vi "Power up time PWM rw.vi"(5 "INDEX":enum16{"Read", "Write"}(ring), 7 "IP":string="192.168.23.100", 8 "error in (no error)":errorcluster, 9 "PWR UP TIME(ms)":u16(knob)=5 min=5 max=2000 step=1 scale=5.0..2000.0, 10 "PORT":dbl=1.0 min=1.0 max=4.0 step=1.0, 11 "MASTER":dbl=1.0 min=1.0 max=10.0 step=1.0) -> (0 "error out":errorcluster, 2 "Startup time":u32 format="%^#.10g ms")   [LabVIEW 2022 SP3]
uses:
  <vilib>/NI/Advanced HTTP Client/POST (Buffer).vi
  <vilib>/NI/Advanced HTTP Client/Session.lvclass
panel:
  out "JSON STRING PAYLOAD":string
  # "SMART conn PWM start Read /Write"
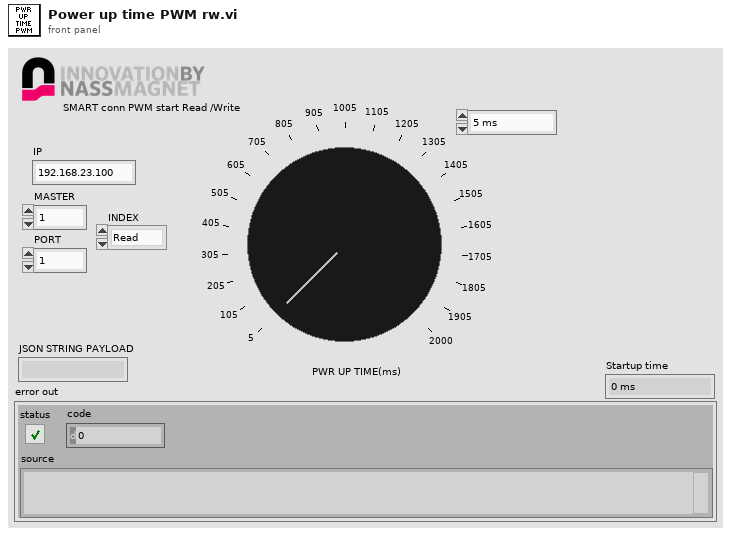
[diagram p1: front panel]
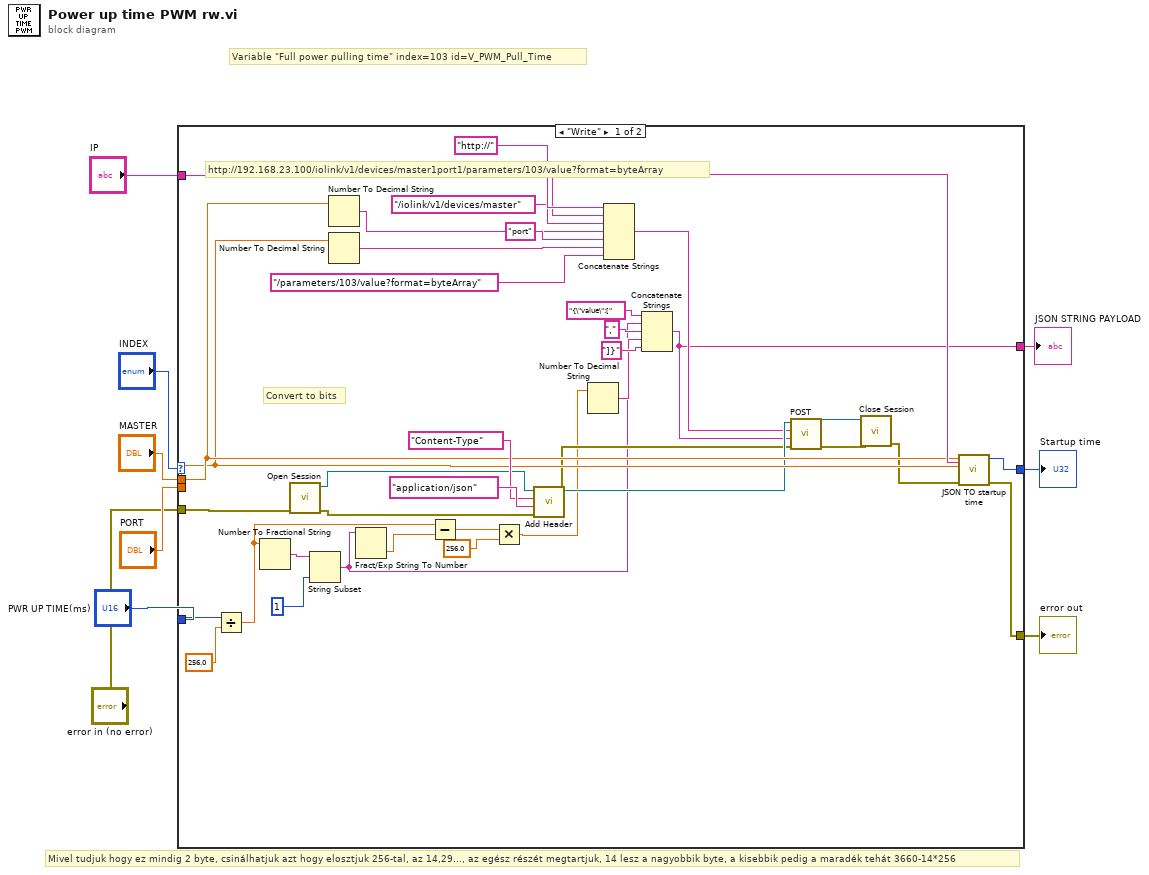
[diagram p0: block diagram]
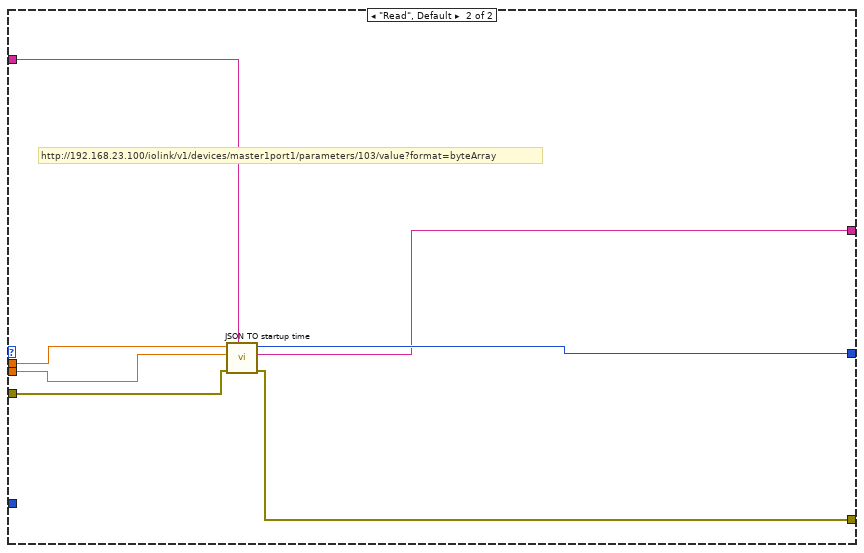
[diagram p2: hidden frame]
diagram:
  # "Variable \"Full power pulling time\" index=103 id=V_PWM_Pull_Time"
  # "Mivel tudjuk hogy ez mindig 2 byte, csinálhatjuk azt hogy elosztjuk 256-tal, az 14,29..., az egész részét megtartjuk, 14 lesz a nagyobbik byte, a kisebbik pedig a maradék tehát 3660-14*256"
  n1 = case shown="\"Write\"" "INDEX" {
    tunnel: "MASTER" -> [w33 w49]
    tunnel: "PORT" -> [w32 w53]
    tunnel: "IP" -> [w36 w52]
    tunnel: [w46 w51] -> w6
    tunnel: [w45 w50] -> w5
    tunnel: "error in (no error)" -> [w41 w48]
    tunnel: [w23 w47] -> w2
    tunnel: "PWR UP TIME(ms)" -> [w21 _]
    frame "Write" {
      # "Convert to bits"
      # "http://192.168.23.100/iolink/v1/devices/master1port1/parameters/103/value?format=byteArray"
      n2 = Divide(x=w21, y=256.0) -> (x/y=w17:dbl)
      n3 = Number To Fractional String(number=w17) -> (F-format string=w20:string)  [unwired: 3 in]
      n4 = call <vilib>:"Open Session.vi"("error in"=w41) -> ("error out"=w40:errorcluster, "session"=w42:refnum<class "Session.lvclass">)  [unwired: 9 in]
      n5 = String Subset(string=w20, length (rest)=1 ("length (rest)")) -> (substring=w18:string)  [unwired: 1 in]
      n6 = Number To Decimal String(number=w33) -> (decimal integer string=w35:string)  [unwired: 1 in]
      n7 = Number To Decimal String(number=w32) -> (decimal integer string=w34:string)  [unwired: 1 in]
      n8 = Fract/Exp String To Number(string=w18) -> (number=w16:dbl)  [unwired: 3 in, 1 out]
      n9 = Subtract(x=w17, y=w16) -> (x-y=w15:dbl)
      n10 = Multiply(x=w15, y=256.0) -> (x*y=w13:dbl)
      n11 = call <vilib>:"Add Header.vi"("error in"=w40, "value"="application/json" ("buffer"), "header"="Content-Type", "session in"=w42) -> ("error out"=w28:errorcluster, "session out"=w30:refnum<class "Session.lvclass">)  [unwired: 6 in]
      n12 = Number To Decimal String(number=w13) -> (decimal integer string=w24:string)  [unwired: 1 in]
      n13 = Concatenate Strings("http://", w36, "/iolink/v1/devices/master" ("string"), w35, "port" ("string"), w34, "/parameters/103/value?format=byteArray" ("string")) -> (w29:string)
      n14 = Concatenate Strings("{\"value\":[" ("data"), w18, "," ("string"), w24, "]}" ("string")) -> (w23:string)
      n15 = call-poly <vilib>:"POST.vi"("error in"=w28, "buffer"=w23, "url"=w29, "session in"=w30) -> ("error out"=w11:errorcluster, "session out"=w12:refnum<class "Session.lvclass">)  [unwired: 3 in, 3 out]
      n16 = call <vilib>:"Close Session.vi"("error in"=w11, "session"=w12) -> ("error out"=w10:errorcluster)  [unwired: 9 in]
      n17 = call "JSON TO startup time.vi"("IP"=w36, "error in (no error)"=w10, "PORT"=w32, "MASTER"=w33) -> ("error out"=w45:errorcluster, "Startup time"=w46:u32)  [unwired: 5 in, 1 out]
    }
    frame "Read", Default {
      # "http://192.168.23.100/iolink/v1/devices/master1port1/parameters/103/value?format=byteArray"
      n18 = call "JSON TO startup time.vi"("IP"=w52, "error in (no error)"=w48, "PORT"=w53, "MASTER"=w49) -> ("error out"=w50:errorcluster, "JSON data"=w47:string, "Startup time"=w51:u32)  [unwired: 5 in]
    }
  }
  "error out" <- w5
  "Startup time" <- w6
  "JSON STRING PAYLOAD" <- w2
